vi "unreserveDevice.vi"(8 "error in (no error)":errorcluster, 10 "deviceName":string, 11 "HWController.lvclass in":refnum<class "HWController.lvclass">) -> (0 "error out":errorcluster, 3 "HWController.lvclass out":refnum<class "HWController.lvclass">)   [LabVIEW 2011, in "Hardware.lvlib" / "HWControllers.lvlib" / "HWController.lvclass"]
doc: "This device is now available for other users"
uses:
  HWController.lvclass
  HWController.lvclass/HWController.ctl
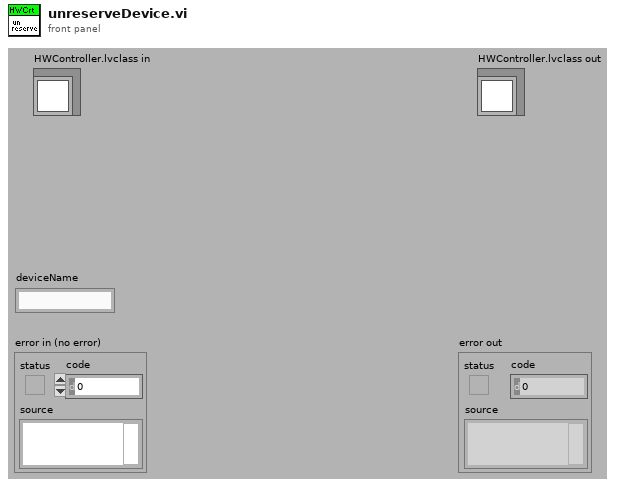
[diagram p1: front panel]
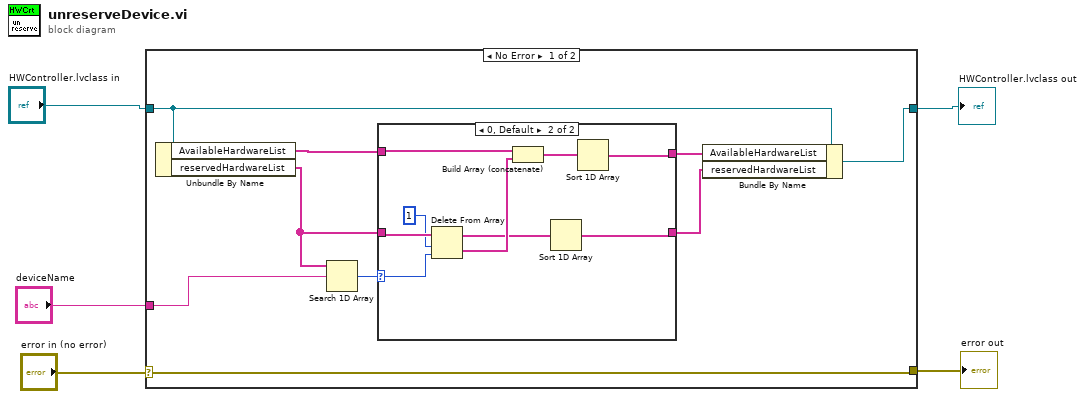
[diagram p0: block diagram]
diagram:
  n1 = case shown="No Error" "error in (no error)" {
    selector: "error in (no error)" -> [w14 w27]
    tunnel: [w14 w27] -> w4
    tunnel: [w6 w26] -> w1
    tunnel: "HWController.lvclass in" -> [w9 w26]
    tunnel: "deviceName" -> [w13 _]
    frame No Error {
      n2 = Unbundle By Name(w9) -> ("AvailableHardwareList"=w10:string[], "reservedHardwareList"=w11:string[])
      n3 = Search 1D Array(1D array=w11, element=w13) -> (index of element=w12:i32)  [unwired: 1 in]
      n4 = case shown="0, Default" w12 {
        selector: w12 -> [_ w23]
        tunnel: w11 -> [w16 w25]
        tunnel: [w16 w19] -> w7
        tunnel: w10 -> [w15 w22]
        tunnel: [w15 w17] -> w8
        frame -1 {
        }
        frame 0, Default {
          n5 = Delete From Array(array=w25, length=1, index=w23) -> (deleted portion=w21:string[], array with subset deleted=w20:string[])
          n6 = Build Array (concatenate)(w22, w21) -> (w18:string[])
          n7 = Sort 1D Array(array=w20) -> (sorted array=w19:string[])
          n8 = Sort 1D Array(array=w18) -> (sorted array=w17:string[])
        }
      }
      n9 = Bundle By Name(cluster=w9, "AvailableHardwareList"=w8, "reservedHardwareList"=w7) -> (w6:refnum<class "HWController.lvclass">)
    }
    frame Error {
    }
  }
  "error out" <- w4
  "HWController.lvclass out" <- w1
